vi "TestView_Tree_Single_ConfigFP.vi"(0 "reference in":refnum<class "TestView_Tree_Single.lvclass">, 5 "error in (no error)":errorcluster) -> (14 "reference out":refnum<class "TestView_Tree_Single.lvclass">, 19 "error out":errorcluster)   [LabVIEW 2022 SP3, in "TestView_Tree_Single.lvlib" / "TestView_Tree_Single.lvclass"]
uses:
  TestView_Tree_Single.lvclass
  protected/Config.ctl
  Components/ViPER.lvlibp/ViPER.lvclass
  C:/Projects/Medulla/ViPER/Examples/Flux_Capacitor_Tester/Components/ViPER.lvlibp/ViPER.lvclass
panel:
  in  "Config":T1
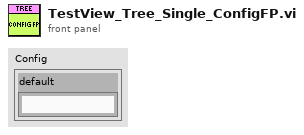
[diagram p1: front panel]
types:
  T1 = typedef "TestView_Tree_Single.lvlib/TestView_Tree_Single.lvclass/Config.ctl" = cluster{"default":string}
  T2 = enum32{"Invalid", "Standard", "Closed", "Hidden", "Minimized", "Maximized"}
  T3 = typedef "TestView_Tree_Single.lvlib/TestView_Tree_Single.lvclass/ObjectAttributes.ctl" = cluster{"Front Panel":refnum<vi>, "Last_Item":string, "Config":T1, "Title":string, "User":string, "TreeRef":refnum<vi>, "Active DUT":i32, "Status":T4, "SN":string, "Spec":string}
  T4 = typedef "TestView_Base.lvlibp/TestView_Base.lvclass/ViewStatus.ctl" = enum16{"Testing", "Ready", "Logout", "Login", "PASS", "FAIL", "FAULT", "ABORTED"}
  T5 = typedef "LVRectTypeDef.ctl" = cluster{"Left":i16, "Top":i16, "Right":i16, "Bottom":i16}
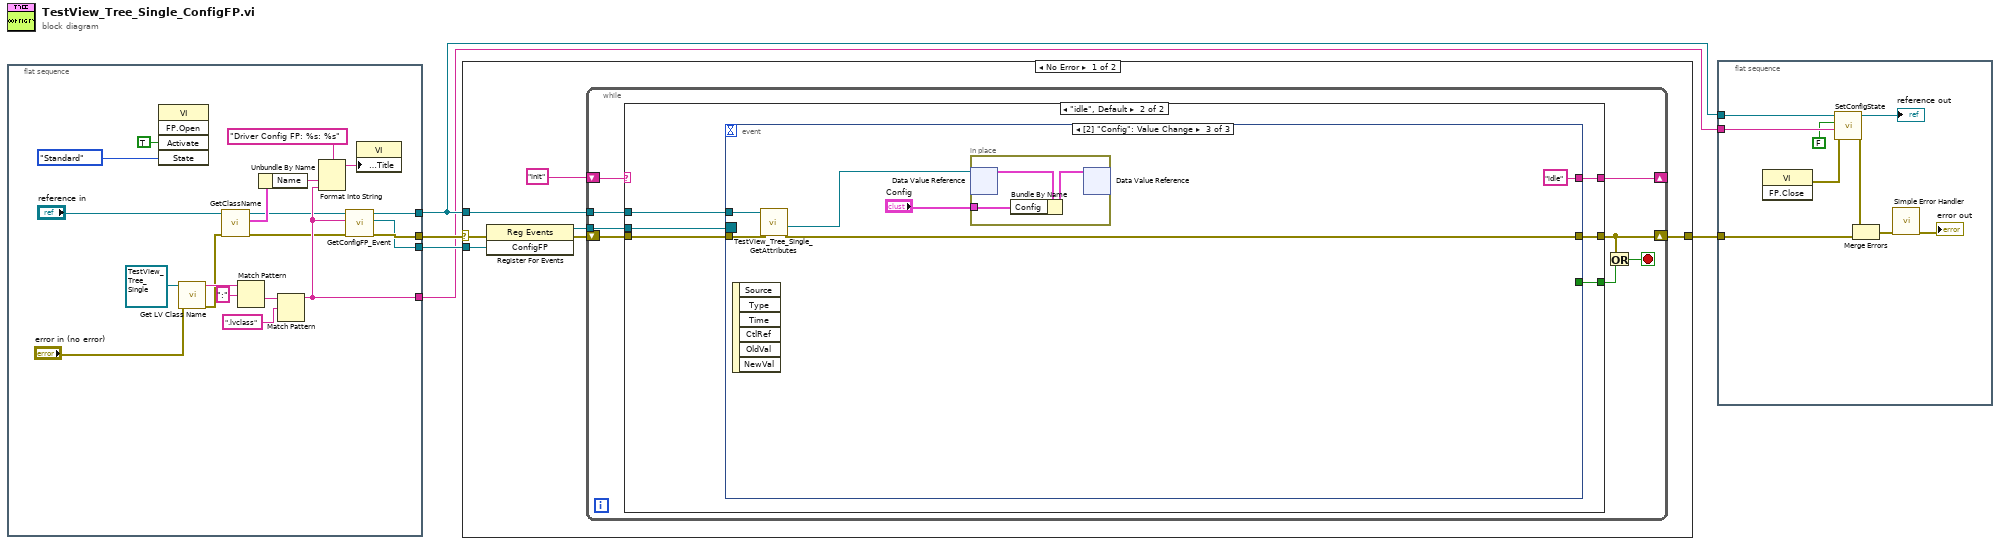
[diagram p0: block diagram]
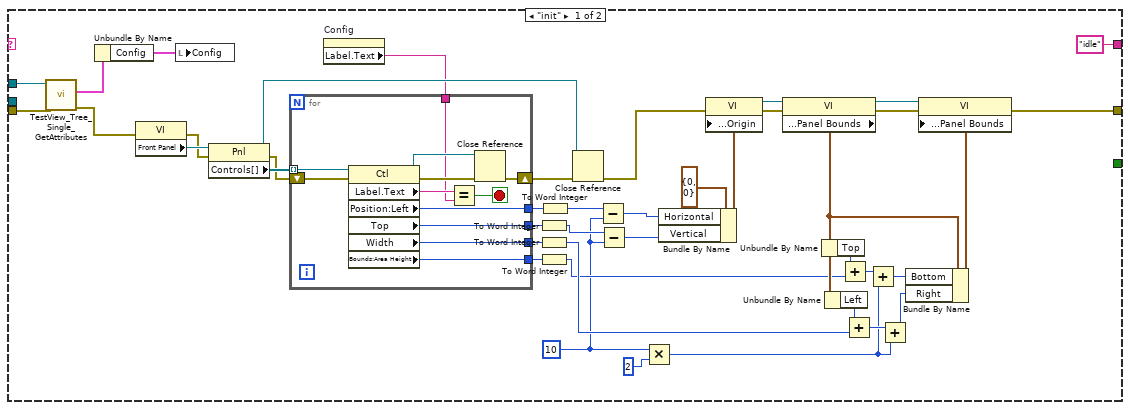
[diagram p2: hidden frame]
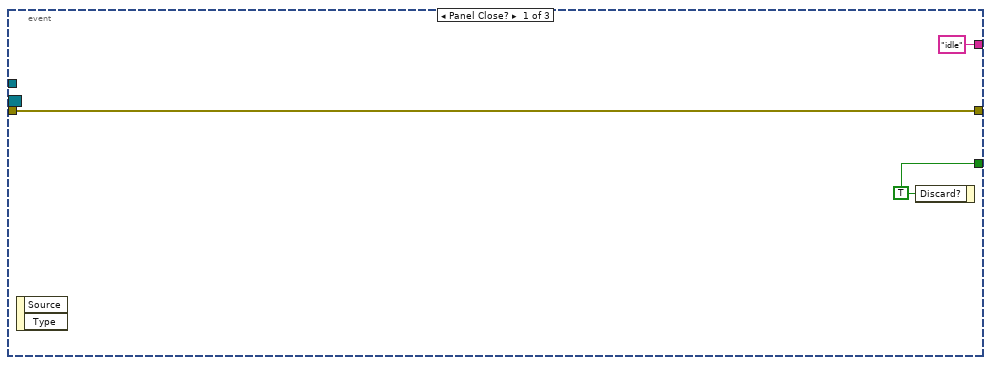
[diagram p3: hidden frame]
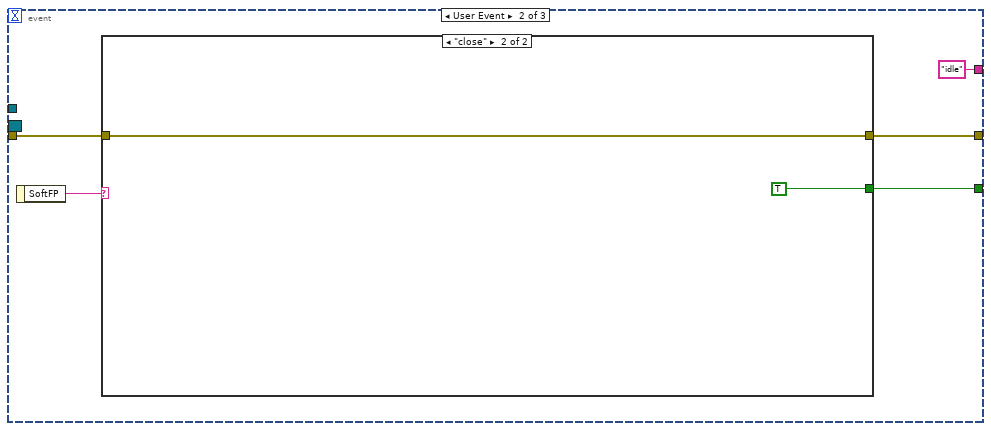
[diagram p4: hidden frame]
diagram:
  n1 = flat-sequence {
    tunnel: [w21] -> w5
    tunnel: [w22] -> w2
    tunnel: [w20] -> w3
    tunnel: [w14] -> w1
    frame #0 {
      n2 = invoke class="VI" method="FP.Open"("Activate"=TRUE ("Activate?"), "State"=T2."Standard") -> ()  [unwired: 3 in, 5 out]
      n3 = call <vilib>:"Get LV Class Name.vi"("error in (no error)"="error in (no error)", "object"=refnum<class "TestView_Tree_Single.lvclass"> refnum ("TestView_Tree.lvlib:TestView_Tree")) -> ("error out"=w12:errorcluster, "class name"=w18:string)  [unwired: 8 in]
      n4 = call "GetClassName.vi"("error in (no error)"=w12, "reference in"="reference in") -> ("error out"=w11:errorcluster, "Details"=w10:cluster{"Name":string, "Class":string}, "reference out"=w9:refnum<class "TestView_Tree_Single.lvclass">)  [unwired: 7 in]
      n5 = Match Pattern(string=w18, regular expression=":") -> (after substring=w17:string)  [unwired: 1 in, 3 out]
      n6 = Unbundle By Name(w10) -> ("Name"=w23:string)
      n7 = Match Pattern(string=w17, regular expression=".lvclass") -> (before substring=w14:string)  [unwired: 1 in, 3 out]
      n8 = Format Into String(format string="Driver Config FP: %s: %s", w23, w14) -> (resulting string=w25:string)  [unwired: 2 in, 1 out]
      n9 = call-dynamic "GetConfigFP_Event.vi"("error in (no error)"=w11, "Ancestor"=w14, "reference in"=w9) -> ("error out"=w21:errorcluster, "ConfigFP"=w20:refnum<user-event>, "reference out"=w22:refnum<class "TestView_Tree_Single.lvclass">)  [unwired: 6 in]
      n10 = property class="VI"("Front Panel.Title"=w25) -> ()  [unwired: 2 in, 2 out]
    }
  }
  n11 = case shown="No Error" w5 {
    selector: w5 -> [w30 w121]
    tunnel: [w26 w121] -> w4
    tunnel: w2 -> [w27 _]
    tunnel: w3 -> [w32 _]
    frame No Error {
      n12 = register-events(error in=w30, w32) -> (reference out=w31:refnum<event-registration>, error out=w29:errorcluster)  [unwired: 1 in]
      n13 = while {
        shift-right: [w37] -> w26
        shift-left: w29 -> [w40]
        tunnel: w31 -> [w39]
        tunnel: w27 -> [w38]
        shift-right: [w33] -> _
        shift-left: "init" -> [w34]
        stop <- w36 stop-if-true
        n14 = case shown="\"idle\", Default" w34 {
          tunnel: w40 -> [w44 w100]
          tunnel: w39 -> [_ w99]
          tunnel: w38 -> [w43 w98]
          tunnel: [w47 w97] -> w37
          tunnel: [_ w96] -> w35
          tunnel: ["idle" w95] -> w33
          frame "init" {
            w48 = i16 10 ("16bit integer")
            n15 = call "TestView_Tree_Single_GetAttributes.vi"("error in (no error)"=w44, "reference in"=w43) -> ("error out"=w42:errorcluster, "Data"=w41:T3)  [unwired: 6 in, 2 out]
            n16 = Unbundle By Name(w41) -> ("Config"=w81:T1)
            n17 = property on="Property Node" class="VI"(error in=w42) -> (error out=w78:errorcluster, "Front Panel"=w80:refnum<vi>)  [unwired: 1 in, 1 out]
            n18 = local write "Config"(w81) -> ()
            n19 = property on="Property Node" class="Pnl"(reference=w80, error in=w78) -> (reference out=w53:refnum<vi>, error out=w77:errorcluster, "Controls[]"=w79:refnum<vi>[])
            n20 = property on="Config" class="Clust (strict)"() -> ("Label.Text"=w45:string)  [unwired: 2 in, 2 out]
            n21 = for {
              tunnel: w79 -> [w94] mode=indexing
              tunnel: [w90] -> w52
              tunnel: [w89] -> w50
              tunnel: [w88] -> w49
              shift-right: [w85] -> w54
              shift-left: w77 -> [w91]
              tunnel: [w87] -> w51
              tunnel: w45 -> [w83]
              stop <- w92 stop-if-true
              n22 = property class="Ctl"(reference=w94, error in=w91) -> (reference out=w84:refnum<vi>, error out=w86:errorcluster, "Label.Text"=w93:string, "Position:Left"=w90:i32, "Top"=w87:i32, "Width"=w89:u32, "Bounds:Area Height"=w88:u32)
              n23 = Equal?(x=w93, y=w83) -> (x = y?=w92:bool)
              n24 = Close Reference(reference=w84, error in (no error)=w86) -> (error out=w85:errorcluster)
            }
            n25 = To Word Integer(number=w51) -> (16bit integer=w55:i16)
            n26 = To Word Integer(number=w50) -> (16bit integer=w58:i16)
            n27 = To Word Integer(number=w49) -> (16bit integer=w57:i16)
            n28 = To Word Integer(number=w52) -> (16bit integer=w56:i16)
            n29 = Close Reference(reference=w53, error in (no error)=w54) -> (error out=w46:errorcluster)
            n30 = Subtract(x=w56, y=w48) -> (x-y=w65:i16)
            n31 = Subtract(x=w55, y=w48) -> (x-y=w66:i16)
            n32 = Multiply(x=w48, y=i16 2) -> (x*y=w59:i16)
            n33 = Bundle By Name(cluster=cluster{"Horizontal":i16, "Vertical":i16} {"Horizontal"=0, "Vertical"=0} ("Front Panel Window:Origin"), "Horizontal"=w65, "Vertical"=w66) -> (w63:cluster{"Horizontal":i16, "Vertical":i16})
            n34 = property on="Property Node" class="VI"(error in=w46, "Front Panel Window:Origin"=w63) -> (reference out=w75:refnum<vi>, error out=w61:errorcluster)  [unwired: 1 in]
            n35 = property on="Property Node" class="VI"(reference=w75, error in=w61) -> (reference out=w76:refnum<vi>, error out=w60:errorcluster, "Front Panel Window:Panel Bounds"=w67:T5)
            n36 = Unbundle By Name(w67) -> ("Top"=w68:i16)
            n37 = Unbundle By Name(w67) -> ("Left"=w69:i16)
            n38 = Add(x=w68, y=w57) -> (x+y=w73:i16)
            n39 = Add(x=w69, y=w58) -> (x+y=w71:i16)
            n40 = Add(x=w73, y=w59) -> (x+y=w74:i16)
            n41 = Add(x=w71, y=w59) -> (x+y=w72:i16)
            n42 = Bundle By Name(cluster=w67, "Bottom"=w74, "Right"=w72) -> (w70:T5)
            n43 = property on="Property Node" class="VI"(reference=w76, error in=w60, "Front Panel Window:Panel Bounds"=w70) -> (error out=w47:errorcluster)  [unwired: 1 out]
          }
          frame "idle", Default {
            n44 = event shown="[2] \"Config\": Value Change" {
              selector: w99 -> [_ _ _]
              dyn-events: _ -> [_ _ _]
              timeout: _ -> [_ _ _]
              tunnel: w100 -> [w103 w108 w115]
              tunnel: [w103 w106 w114] -> w97
              tunnel: [w102 w105 _] -> w96
              tunnel: w98 -> [_ _ w112]
              tunnel: ["idle" "idle" "idle"] -> w95
              event Panel Close? {
                w102 = TRUE ("Discard?")
                n45 = event-data() -> ()  [unwired: 1 in, 2 out]
                n46 = event-data("Discard?"=w102) -> ()  [unwired: 1 in, 1 out]
              }
              event User Event {
                n47 = event-data() -> ("SoftFP"=w107:string)  [unwired: 1 in]
                n48 = case shown="\"close\"" w107 {
                  tunnel: w108 -> [w109 w111]
                  tunnel: [w109 w111] -> w106
                  tunnel: [_ TRUE ("Discard?")] -> w105
                  frame Default {
                  }
                  frame "close" {
                  }
                }
              }
              event Value Change {
                n49 = event-data() -> ()  [unwired: 1 in, 6 out]
                n50 = call "TestView_Tree_Single_GetAttributes.vi"("error in (no error)"=w115, "reference in"=w112) -> ("error out"=w114:errorcluster, "DataRef"=w113:refnum<data-value>)  [unwired: 6 in, 2 out]
                n51 = in-place {
                  in-place-border: "Config" -> [w118]
                  n52 = in-place-dvr #1(w113) -> (w120:T3)  [unwired: 1 out]
                  n53 = Bundle By Name(cluster=w120, "Config"=w118) -> (w119:T3)
                  n54 = in-place-dvr #1(w119) -> ()  [unwired: 2 out]
                }
              }
            }
          }
        }
        n55 = Or(x=w37, y=w35) -> (x .or. y?=w36:bool)
      }
    }
    frame Error {
    }
  }
  n56 = flat-sequence {
    tunnel: w4 -> [w128]
    tunnel: w2 -> [w124]
    tunnel: w1 -> [w126]
    frame #0 {
      n57 = invoke class="VI" method="FP.Close"() -> (error out=w127:errorcluster)  [unwired: 3 in, 2 out]
      n58 = call "SetConfigState.vi"("error in (no error)"=w127, "Ancestor"=w126, "Config Open"=FALSE ("SP Open"), "reference in"=w124) -> ("error out"=w123:errorcluster, "reference out"=→"reference out":refnum<class "TestView_Tree_Single.lvclass">)  [unwired: 6 in]
      n59 = Merge Errors(w123, w128) -> (w130:errorcluster)
      n60 = call <vilib>:"Simple Error Handler.vi"("error in (no error)"=w130) -> ("error out"=→"error out":errorcluster)  [unwired: 4 in, 4 out]
    }
  }
